vi "preposttrigger.vi"(6 "Trigger line":u32(ring) items=["External trigger 0", "External trigger 1", "External trigger 2", "External trigger 3", "RTSI line 0", "RTSI line 1", "RTSI line 2", "RTSI line 3", "RTSI line 4", "RTSI line 5", "RTSI line 6"], 8 "File Path":string="c:\\images\\", 10 "Post-Trigger Images":u32=5, 11 "Pre-Trigger Images":u32=5) -> ()   [LabVIEW 2018]
panel:
  in  "Trigger Polarity":bool
  out "Last Valid Frame":i32
  in  "Interface Name":string="img0"
  # "This example acquires a specified number of pre-trigger and post-trigger\nimages and then saves them to disk as a bitmap. The trigger line can be\nany available external trigger lines or a RTSI line.\n\nNote:  This example requires IMAQ Vision."
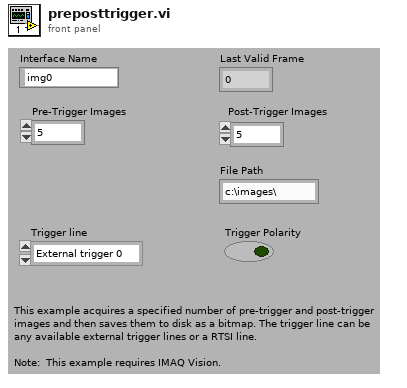
[diagram p1: front panel]
types:
  T1 = typedef "IMAQ Image.ctl" = refnum<image>
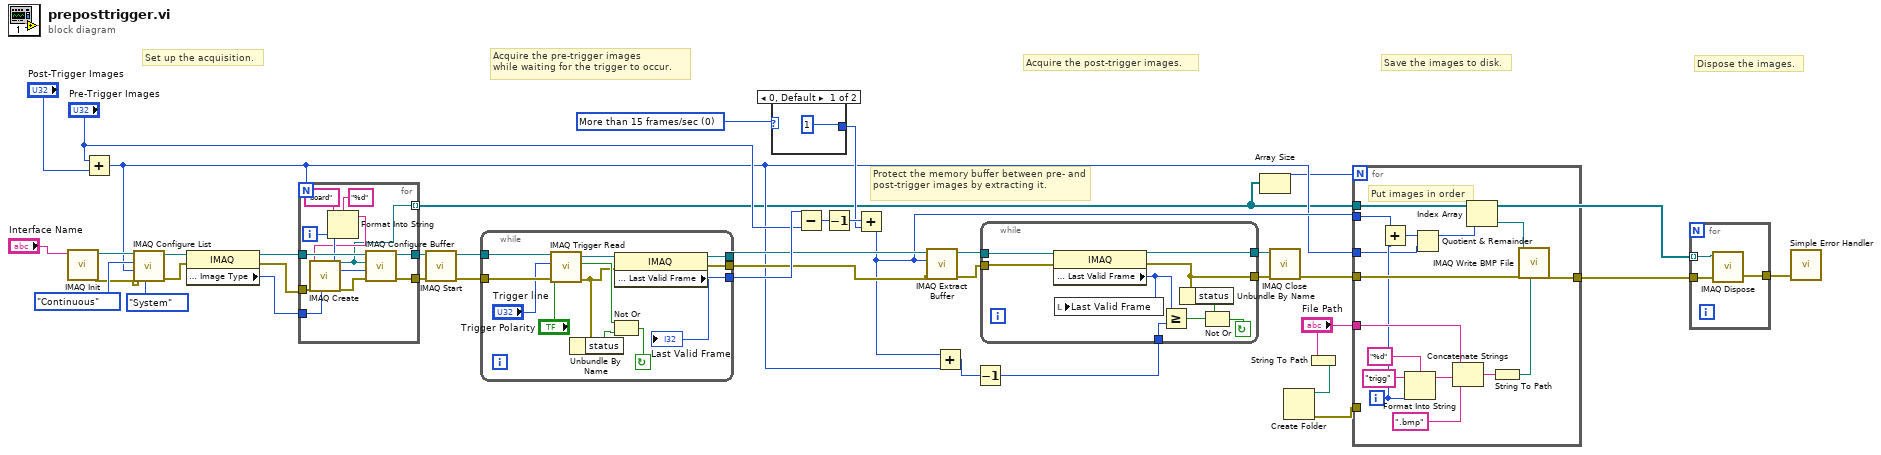
[diagram p0: block diagram]
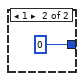
[diagram p2: hidden frame]
diagram:
  w16 = u16 0 items=["More than 15 frames/sec", "15 frames/sec or less"] ("Frame Rate")
  # "Dispose the images."
  # "Save the images to disk."
  # "Protect the memory buffer between pre- and post-trigger images by extracting it."
  # "Acquire the post-trigger images."
  # "Acquire the pre-trigger images \nwhile waiting for the trigger to occur."
  # "Set up the acquisition."
  n1 = call <vilib>:"IMAQ Init.vi"("Interface Name"="Interface Name") -> ("error out"=w36:errorcluster, "IMAQ Session Out"=w39:refnum<k11>)  [unwired: 9 in]
  n2 = Add(x="Pre-Trigger Images", y="Post-Trigger Images") -> (x+y=w3:u32)
  n3 = call <vilib>:"IMAQ Configure List.vi"("Memory Location"=enum16{"System", "Onboard"}."System", "error in (no error)"=w36, "Number of buffers"=w3, "Continuous?"=enum16{"One-Shot", "Continuous"}."Continuous" ("Continuous ?"), "IMAQ Session In"=w39) -> ("error out"=w31:errorcluster, "IMAQ Session Out"=w32:refnum<k11>)  [unwired: 5 in]
  n4 = property class="IMAQ"(reference=w32, error in=w31) -> (reference out=w19:refnum<k11>, error out=w13:errorcluster, "Image Parameters : Image Type"=w30:u32)
  n5 = for {
    N: w3 -> [_]
    tunnel: [w50] -> w34
    tunnel: [w49] -> w35
    tunnel: w19 -> [w48]
    tunnel: w13 -> [w46]
    tunnel: w30 -> [w41]
    tunnel: [w40] -> w2 mode=indexing
    i -> [w43]
    n6 = Format Into String(format string="%d", initial string="board", w43) -> (resulting string=w42:string)  [unwired: 1 in, 1 out]
    n7 = call "IMAQ Create"("Image Name"=w42, "Image Type"=w41, "error in (no error)"=w46) -> ("New Image"=w40:T1, "error out"=w47:errorcluster)  [unwired: 2 in]
    n8 = call <vilib>:"IMAQ Configure Buffer.vi"("error in (no error)"=w47, "Buffer Number"=w43, "Image In"=w40, "IMAQ Session In"=w48) -> ("error out"=w49:errorcluster, "IMAQ Session Out"=w50:refnum<k11>)  [unwired: 6 in]
  }
  n9 = call <vilib>:"IMAQ Start.vi"("error in (no error)"=w35, "IMAQ Session In"=w34) -> ("error out"=w28:errorcluster, "IMAQ Session Out"=w29:refnum<k11>)  [unwired: 8 in]
  n10 = while {
    tunnel: w29 -> [w60]
    tunnel: w28 -> [w59]
    tunnel: [w62] -> w20
    tunnel: [w61] -> w6
    tunnel: [w58] -> w22
    stop <- w51 continue-if-true
    n11 = call <vilib>:"IMAQ Trigger Read.vi"("error in (no error)"=w59, "Polarity"="Trigger Polarity", "Trigger line"="Trigger line", "IMAQ Session In"=w60) -> ("error out"=w53:errorcluster, "Trigger status"=w54:bool, "IMAQ Session Out"=w57:refnum<k11>)  [unwired: 5 in]
    n12 = Unbundle By Name(w53) -> ("status"=w52:bool)
    n13 = Not Or(1:w52, 2:w54) -> (0:w51:bool)
    n14 = property class="IMAQ"(reference=w57, error in=w53) -> (reference out=w62:refnum<k11>, error out=w61:errorcluster, "Status Information : Last Valid Frame"=w58:u32)
    "Last Valid Frame" <- w58
  }
  n15 = case shown="0, Default" w16 {
    tunnel: [1 0] -> w15
    frame 0, Default {
    }
    frame 1 {
    }
  }
  n16 = Subtract(x=w22, y="Pre-Trigger Images") -> (x-y=w25:u32)
  n17 = Decrement(x=w25) -> (x-1=w18:u32)
  n18 = Add(x=w18, y=w15) -> (x+y=w4:u32)
  n19 = call <vilib>:"IMAQ Extract Buffer.vi"("error in (no error)"=w6, "Buffer to extract"=w4, "IMAQ Session In"=w20) -> ("error out"=w5:errorcluster, "IMAQ Session Out"=w17:refnum<k11>)  [unwired: 3 in, 4 out]
  n20 = Add(x=w4, y=w3) -> (x+y=w24:u32)
  n21 = Decrement(x=w24) -> (x-1=w23:u32)
  n22 = while {
    tunnel: w17 -> [w73]
    tunnel: w5 -> [w72]
    tunnel: [w71] -> w27
    tunnel: [w68] -> w26
    tunnel: w23 -> [w70]
    stop <- w65 continue-if-true
    n23 = property class="IMAQ"(reference=w73, error in=w72) -> (reference out=w71:refnum<k11>, error out=w68:errorcluster, "Status Information : Last Valid Frame"=w69:u32)
    n24 = local write "Last Valid Frame"(w69) -> ()
    n25 = Greater Or Equal?(x=w69, y=w70) -> (x >= y?=w66:bool)
    n26 = Unbundle By Name(w68) -> ("status"=w67:bool)
    n27 = Not Or(1:w66, 2:w67) -> (0:w65:bool)
  }
  n28 = Array Size(array=w2) -> (size(s)=w1:i32)
  n29 = call <vilib>:"IMAQ Close.vi"("error in (no error)"=w26, "IMAQ Session In"=w27) -> ("error out"=w11:errorcluster)  [unwired: 9 in]
  n30 = String To Path(string="File Path") -> (path=w8:path)
  n31 = Create Folder(path (use dialog)=w8) -> (error out=w7:errorcluster)  [unwired: 2 in, 2 out]
  n32 = for {
    N: w1 -> [_]
    tunnel: [w89] -> w10
    tunnel: w2 -> [w80]
    tunnel: w11 -> [w82]
    tunnel: "File Path" -> [w81]
    tunnel: w7 -> [_]
    tunnel: w4 -> [w78]
    tunnel: w3 -> [w76]
    i -> [w79]
    # "Put images in order"
    n33 = Add(x=w78, y=w79) -> (x+y=w77:u32)
    n34 = Format Into String(format string="%d", initial string="trigg", w79) -> (resulting string=w86:string)  [unwired: 1 in, 1 out]
    n35 = Quotient & Remainder(x=w77, y=w76) -> (x-y*floor(x/y)=w75:u32)  [unwired: 1 out]
    n36 = Concatenate Strings(w81, w86, ".bmp") -> (w84:string)
    n37 = Index Array(array=w80, index=w75) -> (element=w74:T1)
    n38 = String To Path(string=w84) -> (path=w83:path)
    n39 = call "IMAQ Write BMP File"("error in (no error)"=w82, "File Path"=w83, "Image"=w74) -> ("error out"=w89:errorcluster)  [unwired: 5 in]
  }
  n40 = for {
    tunnel: [w92] -> w14
    tunnel: w10 -> [w91]
    tunnel: w2 -> [w90] mode=indexing
    n41 = call "IMAQ Dispose"("Image"=w90, "error in (no error)"=w91) -> ("error out"=w92:errorcluster)  [unwired: 4 in]
  }
  n42 = call <vilib>:"Simple Error Handler.vi"("error in (no error)"=w14) -> ()  [unwired: 4 in, 5 out]
